vi "RawTest.vi"   [LabVIEW 2016, in "Laser Diode Controller.lvlib" / "Laser Diode Controller.lvclass"]
uses:
  Laser Diode Controller.lvclass
  C:/Data/SVN/Projects/IDEXX/ProCyte Laser Fixture Software/Software/Collimation/data/Thorlabs.MotionControl.KCube.LaserDiodeCLI.dll
  data/Thorlabs.MotionControl.KCube.LaserDiodeCLI.dll
  C:/Data/SVN/Projects/IDEXX/ProCyte Laser Fixture Software/Software/Collimation/data/Thorlabs.MotionControl.DeviceManagerCLI.dll
  data/Thorlabs.MotionControl.DeviceManagerCLI.dll
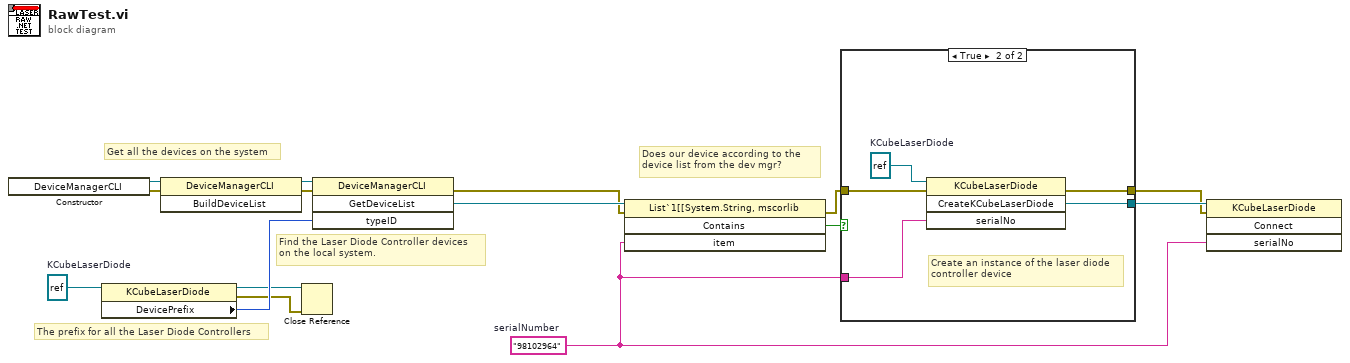
[diagram p0: block diagram]
diagram:
  w1 = "98102964"  # serialNumber
  w11 = refnum<k24> refnum  # KCubeLaserDiode
  # "Does our device according to the \ndevice list from the dev mgr?"
  # "Get all the devices on the system"
  # "The prefix for all the Laser Diode Controllers"
  # "Find the Laser Diode Controller devices\non the local system."
  n1 = constructor class="DeviceManagerCLI"() -> (reference out=w15:refnum<k24>, error out=w14:errorcluster)  [unwired: 3 in, 1 out]
  n2 = property class="KCubeLaserDiode"(reference=w11) -> (reference out=w9:refnum<k24>, error out=w8:errorcluster, "DevicePrefix"=w10:i32)  [unwired: 1 in]
  n3 = invoke class="DeviceManagerCLI" method="BuildDeviceList"(reference=w15, error in=w14) -> (reference out=w13:refnum<k24>, error out=w12:errorcluster)  [unwired: 1 in, 1 out]
  n4 = Close Reference(reference=w9, error in (no error)=w8) -> ()  [unwired: 1 out]
  n5 = invoke class="DeviceManagerCLI" method="GetDeviceList"(reference=w13, error in=w12, "typeID"=w10) -> (error out=w6:errorcluster, "GetDeviceList"=w7:refnum<k24>)  [unwired: 1 in, 2 out]
  n6 = invoke class="List`1[[System.String, mscorlib" method="Contains"(reference=w7, error in=w6, "item"=w1) -> (error out=w4:errorcluster, "Contains"=w5:bool)  [unwired: 1 in, 2 out]
  n7 = case shown="True" w5 {
    tunnel: [w16 w18] -> w2
    tunnel: w4 -> [w16 w21]
    tunnel: w1 -> [_ w19]
    tunnel: [_ w17] -> w3
    frame False {
    }
    frame True {
      w20 = refnum<k24> refnum  # KCubeLaserDiode
      # "Create an instance of the laser diode\ncontroller device"
      n8 = invoke class="KCubeLaserDiode" method="CreateKCubeLaserDiode"(reference=w20, error in=w21, "serialNo"=w19) -> (error out=w18:errorcluster, "CreateKCubeLaserDiode"=w17:refnum<k24>)  [unwired: 1 in, 2 out]
    }
  }
  n9 = invoke class="KCubeLaserDiode" method="Connect"(reference=w3, error in=w2, "serialNo"=w1) -> ()  [unwired: 1 in, 4 out]
